vi "Add Test Suite.vi"(8 "error in (no error)":errorcluster, 10 "Test Suite":refnum<class "Test Suite.lvclass">, 11 "Test Suites in":refnum<class "Test Suites.lvclass">) -> (0 "error out":errorcluster, 3 "Test Suites out":refnum<class "Test Suites.lvclass">)   [LabVIEW 2013, in "JUnit XML.lvlib" / "Test Suites.lvclass"]
doc: "Adds a test suite to the collection."
uses:
  Test Suites.lvclass
  Test Suite/Test Suite.lvclass
  Test Suites.lvclass/Test Suites.ctl
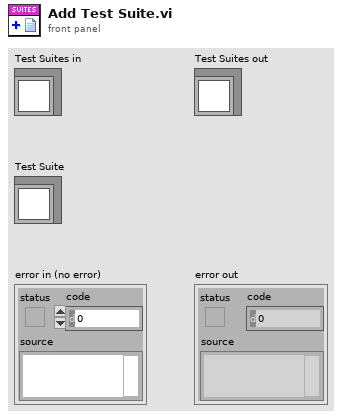
[diagram p1: front panel]
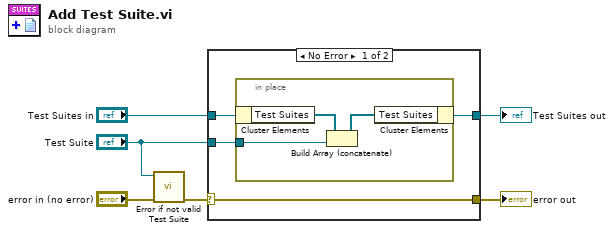
[diagram p0: block diagram]
diagram:
  n1 = call "Error if not valid Test Suite.vi"("error in (no error)"="error in (no error)", "Test Suite"="Test Suite") -> ("error out"=w2:errorcluster)  [unwired: 9 in]
  n2 = case shown="No Error" w2 {
    selector: w2 -> [w10 w15]
    tunnel: [w10 w15] -> w6
    tunnel: [w8 w14] -> w4
    tunnel: "Test Suites in" -> [w9 w14]
    tunnel: "Test Suite" -> [w7 _]
    frame No Error {
      n3 = in-place {
        in-place-border: w7 -> [w12]
        n4 = in-place-cluster #1(w9) -> ("Test Suites"=w13:refnum<class "Test Suite.lvclass">[])
        n5 = Build Array (concatenate)(w13, w12) -> (w11:refnum<class "Test Suite.lvclass">[])
        n6 = in-place-cluster #1("Test Suites"=w11) -> (w8:refnum<class "Test Suites.lvclass">)
      }
    }
    frame Error {
    }
  }
  "error out" <- w6
  "Test Suites out" <- w4
